vi "Home Caller.vi"   [LabVIEW 2020, in "Endigit.lvlib"]
doc: "Places the origin of the front panel of the calling VI at the top left of the panel.\n\nAuthored by Robert C. Mortensen\nrobert@endigit.com\n\nCopyright (c) 2015, Endigit, Inc."
uses:
  Endigit.lvlib
  <vilib>/Utility/miscctls.llb/LVPointTypeDef.ctl
types:
  T1 = typedef "LVPointTypeDef.ctl" = cluster{"Horizontal":i16, "Vertical":i16}
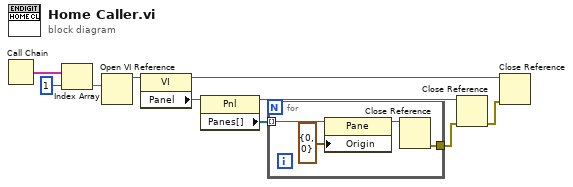
[diagram p0: block diagram]
diagram:
  n1 = Call Chain() -> (call chain=w7:string[])
  n2 = Index Array(array=w7, index=1) -> (element=w6:string)
  n3 = Open VI Reference(vi path=w6) -> (vi reference=w8:refnum<vi>)  [unwired: 5 in, 1 out]
  n4 = property class="VI"(reference=w8) -> (reference out=w2:refnum<vi>, "Panel"=w10:refnum<vi>)  [unwired: 1 in, 1 out]
  n5 = property class="Pnl"(reference=w10) -> (reference out=w4:refnum<vi>, "Panes[]"=w9:refnum<vi>[])  [unwired: 1 in, 1 out]
  n6 = for {
    tunnel: w9 -> [w14] mode=indexing
    tunnel: [w11] -> w3
    n7 = property class="Pane"(reference=w14, "Origin"=T1 {"Horizontal"=0, "Vertical"=0} ("Horizontal Scrollbar Visibility")) -> (reference out=w12:refnum<vi>)  [unwired: 1 in, 1 out]
    n8 = Close Reference(reference=w12) -> (error out=w11:errorcluster)  [unwired: 1 in]
  }
  n9 = Close Reference(reference=w4, error in (no error)=w3) -> (error out=w1:errorcluster)
  n10 = Close Reference(reference=w2, error in (no error)=w1) -> ()  [unwired: 1 out]
